vi "Main.vi"(8 "error in (no error)":errorcluster, 11 "ImageStackBase in":refnum<class "ImageStack.lvclass">) -> (0 "error out":errorcluster, 3 "component":refnum<class "ImageStack.lvclass">)   [LabVIEW 2012, in "ImageStack.lvclass"]
doc: "Main VI of the component."
uses:
  ImageStack.lvclass
  <vilib>/Distrio/Murmex/Murmex/command_enum.ctl
  ImageStack.lvclass/ImageStack.ctl
  <vilib>/Distrio/Murmex/InitialiseMessage/InitialiseMessage.lvclass
  <vilib>/Distrio/Murmex/Murmex/data_compression_enum.ctl
  <vilib>/Distrio/Murmex/TerminateMessage/TerminateMessage.lvclass
  <vilib>/Distrio/Murmex/ConfigureMessage/ConfigureMessage.lvclass
  <vilib>/Distrio/Murmex/Murmex/update_cluster.ctl
  <vilib>/Distrio/Murmex/StartMessage/StartMessage.lvclass
  <vilib>/Distrio/Murmex/StopMessage/StopMessage.lvclass
  <vilib>/Distrio/Murmex/Murmex/Set configure at initialise.vi
  <vilib>/Distrio/Murmex/Murmex/Set log reference.vi
  <vilib>/Distrio/Murmex/Murmex/Set VI reference.vi
  <vilib>/Distrio/Murmex/Murmex/Set relay start stop to observers.vi
  <vilib>/Distrio/Murmex/Murmex/Set data compression.vi
  <vilib>/Distrio/Murmex/Murmex/Set write log to disk.vi
  <vilib>/Distrio/Murmex/Murmex/Murmex.lvclass
  <vilib>/Distrio/Murmex/Message/Message.lvclass
panel:
  in  "button:config":bool
  in  "Tab Control":enum32{"User", "Debug", "About"}(tab)
  in  "button::direction":bool
  in  "File name":string
  out "Translation speed":dbl[unit]
  in  "button:start":bool
  in  "No. of frames":u16=100
  out "Frame rate":dbl[unit]
  in  "Subfolder levels":string[](array[string])
  in  "Step size":dbl[unit]
  out "log":string
  in  "ID":string="stack"
  in  "wait b4 acquisition":dbl[unit]=1.0
  in  "button:send command":bool
  in  "Generic command":string
  in  "command":T1
  in  "button:quit":bool
  in  "terminate?":bool=TRUE
  # "ImageStack\n\nImplemented by:\nLudovico Silvestri\nUniversity of Florence, Italy"
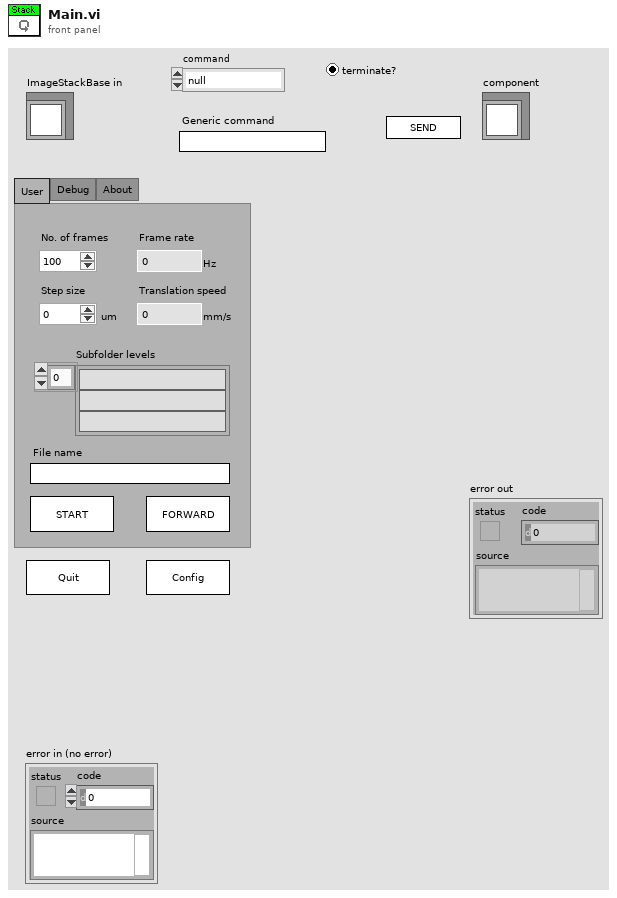
[diagram p1: front panel]
types:
  T1 = typedef "Murmex.lvlib/Murmex.lvclass/command_enum.ctl" = enum16{"null", "initialise", "reset", "terminate", "acknowledge", "update", "inspect", "inform", "proceed", "start", "stop", "fetch", "configure", "generic"}
  T2 = typedef "Murmex.lvlib/Murmex.lvclass/data_compression_enum.ctl" = enum16{"base64", "zip+base64", "byte to string"}
  T3 = typedef "Murmex.lvlib/Murmex.lvclass/update_cluster.ctl" = cluster{"target ID":string, "key chains":string[], "values":variant[]}
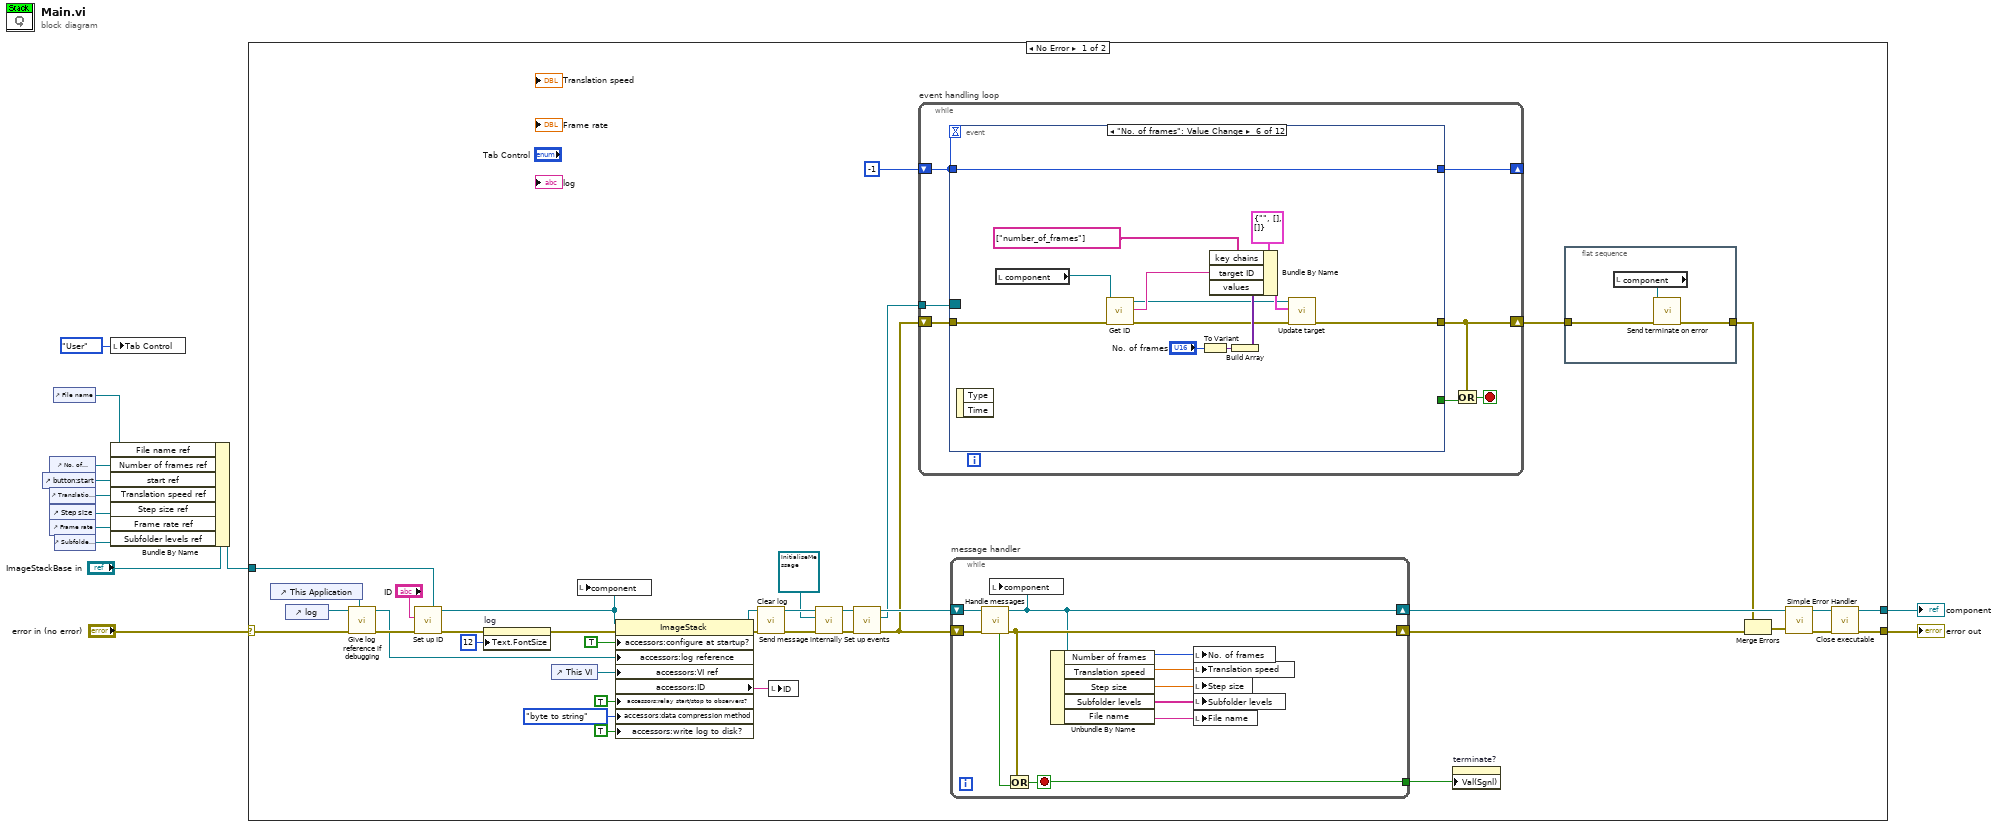
[diagram p0: block diagram]
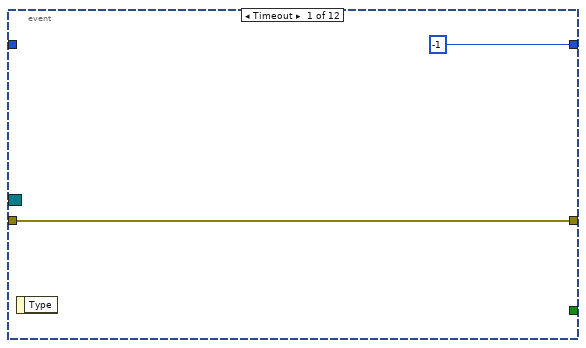
[diagram p2: hidden frame]
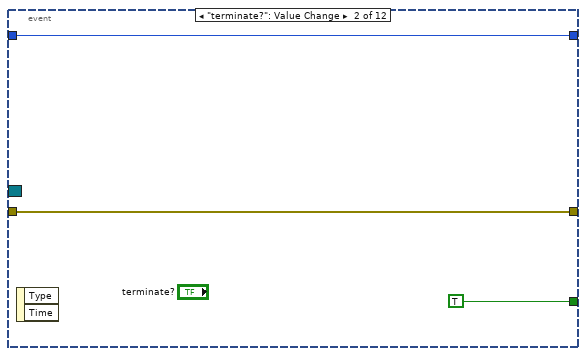
[diagram p3: hidden frame]
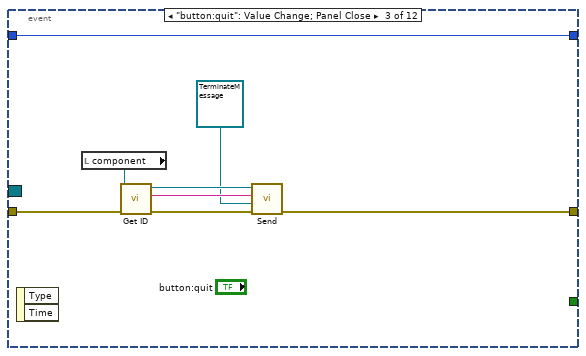
[diagram p4: hidden frame]
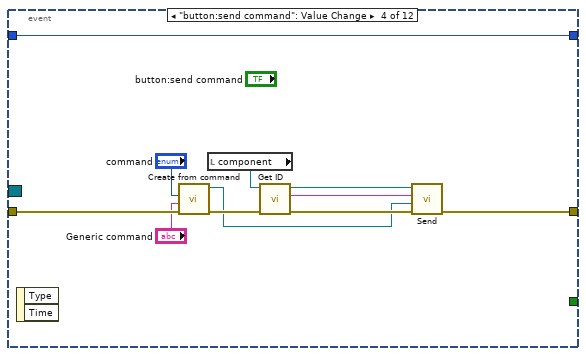
[diagram p5: hidden frame]
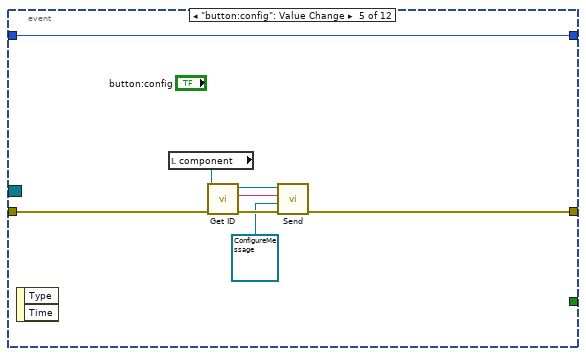
[diagram p6: hidden frame]
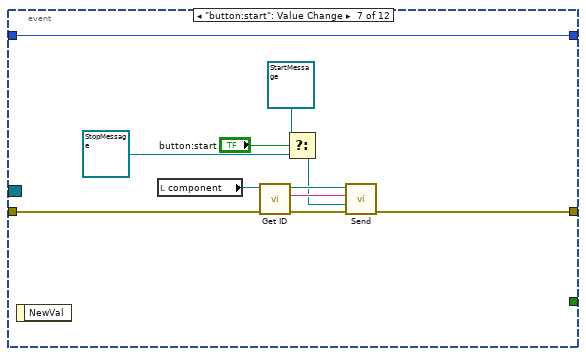
[diagram p7: hidden frame]
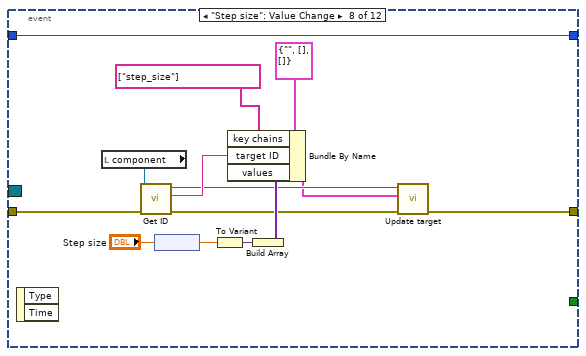
[diagram p8: hidden frame]
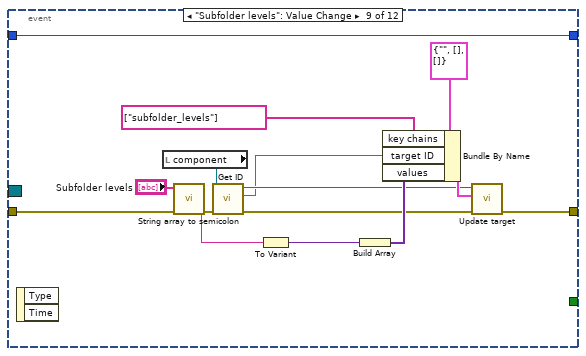
[diagram p9: hidden frame]
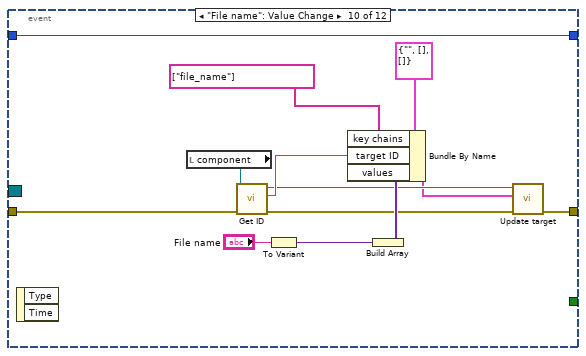
[diagram p10: hidden frame]
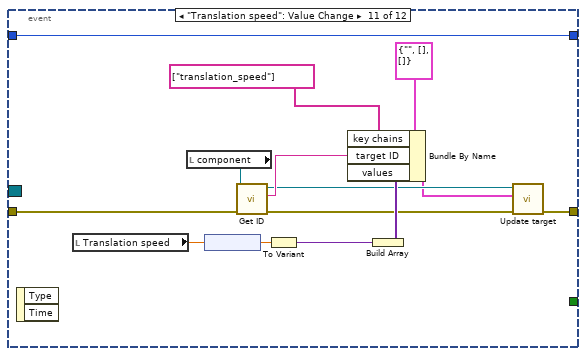
[diagram p11: hidden frame]
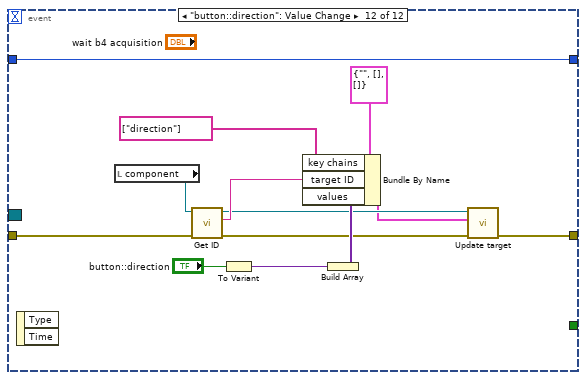
[diagram p12: hidden frame]
diagram:
  n1 = control-ref of="button:start"() -> (w4:refnum<vi>)
  n2 = control-ref of="No. of frames"() -> (w3:refnum<vi>)
  n3 = control-ref of="Translation speed"() -> (w5:refnum<vi>)
  n4 = control-ref of="Step size"() -> (w6:refnum<vi>)
  n5 = control-ref of="Frame rate"() -> (w7:refnum<vi>)
  n6 = control-ref of="File name"() -> (w1:refnum<vi>)
  n7 = control-ref of="Subfolder levels"() -> (w8:refnum<vi>)
  n8 = local write "Tab Control"(enum32{"User", "Debug", "About"}."User" ("Tab Control")) -> ()
  n9 = Bundle By Name(cluster="ImageStackBase in", "File name ref"=w1, "Number of frames ref"=w3, "start ref"=w4, "Translation speed ref"=w5, "Step size ref"=w6, "Frame rate ref"=w7, "Subfolder levels ref"=w8) -> (w9:refnum<class "ImageStack.lvclass">)
  n10 = case shown="No Error" "error in (no error)" {
    selector: "error in (no error)" -> [w19 w197]
    tunnel: w9 -> [w43 w198]
    tunnel: [w22 w198] -> w11
    tunnel: [w23 w197] -> w10
    frame No Error {
      n11 = control-ref of="This Application"() -> (w16:refnum<vi>)
      n12 = control-ref of="log"() -> (w15:refnum<vi>)
      n13 = call "Give log reference if debugging.vi"("application ref"=w16, "error in (no error)"=w19, "log reference in"=w15) -> ("error out"=w18:errorcluster, "log reference out"=w14:refnum<vi>)  [unwired: 6 in, 1 out]
      n14 = call <vilib>:"Set up ID.vi"("error in (no error)"=w18, "component ID"="ID", "MurmexBase in"=w43) -> ("error out"=w32:errorcluster, "MurmexBase out"=w40:refnum<class "ImageStack.lvclass">)  [unwired: 6 in, 1 out]
      n15 = property on="log" class="Str"(error in=w32, "Text.FontSize"=u32 12 ("Text.Font:Size")) -> (error out=w31:errorcluster)  [unwired: 1 in, 1 out]
      n16 = control-ref of="This VI"() -> (w49:refnum<vi>)
      n17 = local write "component"(w40) -> ()
      n18 = property class="ImageStack"(reference=w40, error in=w31, "accessors:configure at startup?"=TRUE ("configure at startup?"), "accessors:log reference"=w14, "accessors:VI ref"=w49, "accessors:relay start/stop to observers?"=TRUE ("relay start/stop to observers?"), "accessors:data compression method"=data_compression_enum."byte to string" ("data compression method"), "accessors:write log to disk?"=TRUE ("write log to disk?")) -> (reference out=w48:refnum<class "ImageStack.lvclass">, error out=w47:errorcluster, "accessors:ID"=w41:string)
      n19 = call <vilib>:"Clear log.vi"("error in (no error)"=w47, "MurmexBase in"=w48) -> ("error out"=w46:errorcluster, "MurmexBase out"=w45:refnum<class "ImageStack.lvclass">)  [unwired: 8 in]
      n20 = local write "ID"(w41) -> ()
      n21 = call <vilib>:"Send message internally.vi"("error in (no error)"=w46, "Message"=refnum<class "InitialiseMessage.lvclass"> refnum ("Murmex.lvlib:InitialiseMessage"), "Murmex in"=w45) -> ("error out"=w39:errorcluster, "Murmex out"=w38:refnum<class "ImageStack.lvclass">)  [unwired: 7 in]
      n22 = call <vilib>:"Set up events.vi"("error in (no error)"=w39, "MurmexBase in"=w38) -> ("error out"=w35:errorcluster, "Event Registration Refnum"=w34:refnum<event-registration>, "MurmexBase out"=w37:refnum<class "ImageStack.lvclass">)  [unwired: 7 in]
      n23 = while "event handling loop" {
        shift-right: [w59] -> _
        shift-left: -1 -> [w60]
        shift-right: [w55] -> w25
        shift-left: w35 -> [w58]
        tunnel: w34 -> [w57]
        stop <- w56 stop-if-true
        n24 = event shown="[5] \"No. of frames\": Value Change" {
          selector: w57 -> [_ _ _ _ _ _ _ _ _ _ _ _]
          dyn-events: _ -> [_ _ _ _ _ _ _ _ _ _ _ _]
          timeout: w60 -> [_ _ _ _ _ _ _ _ _ _ _ _]
          tunnel: w60 -> [_ w63 w66 w74 w85 w101 w106 w118 w140 w148 w162 w173]
          tunnel: [-1 w63 w66 w74 w85 w101 w106 w118 w140 w148 w162 w173] -> w59
          tunnel: [w61 w65 w69 w79 w90 w102 w111 w122 w141 w151 w165 w175] -> w55
          tunnel: w58 -> [w61 w65 w73 w84 w92 w104 w112 w128 w139 w147 w161 w177]
          tunnel: [_ TRUE _ _ _ _ _ _ _ _ _ _] -> w54
          event Timeout {
            n25 = event-data() -> ()  [unwired: 1 in, 1 out]
          }
          event "terminate?": Value Change {
            n26 = event-data() -> ()  [unwired: 1 in, 2 out]
          }
          event "button:quit": Value Change; Panel Close {
            n27 = event-data() -> ()  [unwired: 1 in, 2 out]
            n28 = local read "component"() -> (w72:refnum<class "ImageStack.lvclass">)
            n29 = call <vilib>:"Get ID.vi"("error in (no error)"=w73, "Murmex in"=w72) -> ("error out"=w70:errorcluster, "component id"=w68:string, "Murmex out"=w71:refnum<class "ImageStack.lvclass">)  [unwired: 7 in]
            n30 = call <vilib>:"Send.vi"("error in (no error)"=w70, "Message"=refnum<class "TerminateMessage.lvclass"> refnum ("Murmex.lvlib:TerminateMessage"), "recipient"=w68, "Murmex in"=w71) -> ("error out"=w69:errorcluster)  [unwired: 6 in, 1 out]
          }
          event "button:send command": Value Change {
            n31 = event-data() -> ()  [unwired: 1 in, 2 out]
            n32 = call <vilib>:"Create from command.vi"("error in (no error)"=w84, "generic command"="Generic command", "command"="command") -> ("error out"=w81:errorcluster, "Message out"=w78:refnum<class "Message.lvclass">)  [unwired: 7 in]
            n33 = local read "component"() -> (w77:refnum<class "ImageStack.lvclass">)
            n34 = call <vilib>:"Get ID.vi"("error in (no error)"=w81, "Murmex in"=w77) -> ("error out"=w80:errorcluster, "component id"=w75:string, "Murmex out"=w76:refnum<class "ImageStack.lvclass">)  [unwired: 7 in]
            n35 = call <vilib>:"Send.vi"("error in (no error)"=w80, "Message"=w78, "recipient"=w75, "Murmex in"=w76) -> ("error out"=w79:errorcluster)  [unwired: 6 in, 1 out]
          }
          event "button:config": Value Change {
            n36 = event-data() -> ()  [unwired: 1 in, 2 out]
            n37 = local read "component"() -> (w86:refnum<class "ImageStack.lvclass">)
            n38 = call <vilib>:"Get ID.vi"("error in (no error)"=w92, "Murmex in"=w86) -> ("error out"=w91:errorcluster, "component id"=w88:string, "Murmex out"=w89:refnum<class "ImageStack.lvclass">)  [unwired: 7 in]
            n39 = call <vilib>:"Send.vi"("error in (no error)"=w91, "Message"=refnum<class "ConfigureMessage.lvclass"> refnum ("Murmex.lvlib:ConfigureMessage"), "recipient"=w88, "Murmex in"=w89) -> ("error out"=w90:errorcluster)  [unwired: 6 in, 1 out]
          }
          event "No. of frames": Value Change {
            n40 = event-data() -> ()  [unwired: 1 in, 2 out]
            n41 = local read "component"() -> (w103:refnum<class "ImageStack.lvclass">)
            n42 = call <vilib>:"Get ID.vi"("error in (no error)"=w104, "Murmex in"=w103) -> ("error out"=w93:errorcluster, "component id"=w95:string, "Murmex out"=w94:refnum<class "ImageStack.lvclass">)  [unwired: 7 in]
            n43 = To Variant(anything="No. of frames") -> (Variant=w98:variant)
            n44 = Build Array(w98) -> (w97:variant[])
            n45 = Bundle By Name(cluster=T3 {"target ID"="", "key chains"=[], "values"=[]} ("update cluster"), "key chains"=string[] ["number_of_frames"], "target ID"=w95, "values"=w97) -> (w96:T3)
            n46 = call <vilib>:"Update target.vi"("error in (no error)"=w93, "update cluster"=w96, "MurmexBase in"=w94) -> ("error out"=w102:errorcluster)  [unwired: 7 in, 1 out]
          }
          event "button:start": Value Change {
            n47 = event-data() -> ()  [unwired: 1 in, 1 out]
            n48 = local read "component"() -> (w113:refnum<class "ImageStack.lvclass">)
            n49 = call <vilib>:"Get ID.vi"("error in (no error)"=w112, "Murmex in"=w113) -> ("error out"=w116:errorcluster, "component id"=w114:string, "Murmex out"=w115:refnum<class "ImageStack.lvclass">)  [unwired: 7 in]
            n50 = Select(t=refnum<class "StartMessage.lvclass"> refnum ("Message in"), s="button:start", f=refnum<class "StopMessage.lvclass"> refnum ("Distrio Murmex 1.0:StopMessage")) -> (s? t:f=w108:refnum<class "Message.lvclass">)
            n51 = call <vilib>:"Send.vi"("error in (no error)"=w116, "Message"=w108, "recipient"=w114, "Murmex in"=w115) -> ("error out"=w111:errorcluster)  [unwired: 6 in, 1 out]
          }
          event "Step size": Value Change {
            n52 = event-data() -> ()  [unwired: 1 in, 2 out]
            n53 = local read "component"() -> (w124:refnum<class "ImageStack.lvclass">)
            n54 = call <vilib>:"Get ID.vi"("error in (no error)"=w128, "Murmex in"=w124) -> ("error out"=w123:errorcluster, "component id"=w127:string, "Murmex out"=w121:refnum<class "ImageStack.lvclass">)  [unwired: 7 in]
            n55 = node("Step size") -> (w117:dbl)
            n56 = To Variant(anything=w117) -> (Variant=w126:variant)
            n57 = Build Array(w126) -> (w125:variant[])
            n58 = Bundle By Name(cluster=T3 {"target ID"="", "key chains"=[], "values"=[]} ("update cluster"), "key chains"=string[] ["step_size"], "target ID"=w127, "values"=w125) -> (w120:T3)
            n59 = call <vilib>:"Update target.vi"("error in (no error)"=w123, "update cluster"=w120, "MurmexBase in"=w121) -> ("error out"=w122:errorcluster)  [unwired: 7 in, 1 out]
          }
          event "Subfolder levels": Value Change {
            n60 = event-data() -> ()  [unwired: 1 in, 2 out]
            n61 = local read "component"() -> (w142:refnum<class "ImageStack.lvclass">)
            n62 = call "String array to semicolon.vi"("error in"=w139, "String array"="Subfolder levels") -> ("error out"=w138:errorcluster, "Semicolon string"=w136:string)  [unwired: 8 in]
            n63 = call <vilib>:"Get ID.vi"("error in (no error)"=w138, "Murmex in"=w142) -> ("error out"=w132:errorcluster, "component id"=w131:string, "Murmex out"=w133:refnum<class "ImageStack.lvclass">)  [unwired: 7 in]
            n64 = To Variant(anything=w136) -> (Variant=w143:variant)
            n65 = Build Array(w143) -> (w135:variant[])
            n66 = Bundle By Name(cluster=T3 {"target ID"="", "key chains"=[], "values"=[]} ("update cluster"), "key chains"=string[] ["subfolder_levels"], "target ID"=w131, "values"=w135) -> (w134:T3)
            n67 = call <vilib>:"Update target.vi"("error in (no error)"=w132, "update cluster"=w134, "MurmexBase in"=w133) -> ("error out"=w141:errorcluster)  [unwired: 7 in, 1 out]
          }
          event "File name": Value Change {
            n68 = event-data() -> ()  [unwired: 1 in, 2 out]
            n69 = local read "component"() -> (w153:refnum<class "ImageStack.lvclass">)
            n70 = call <vilib>:"Get ID.vi"("error in (no error)"=w147, "Murmex in"=w153) -> ("error out"=w152:errorcluster, "component id"=w156:string, "Murmex out"=w150:refnum<class "ImageStack.lvclass">)  [unwired: 7 in]
            n71 = To Variant(anything="File name") -> (Variant=w155:variant)
            n72 = Build Array(w155) -> (w154:variant[])
            n73 = Bundle By Name(cluster=T3 {"target ID"="", "key chains"=[], "values"=[]} ("update cluster"), "key chains"=string[] ["file_name"], "target ID"=w156, "values"=w154) -> (w149:T3)
            n74 = call <vilib>:"Update target.vi"("error in (no error)"=w152, "update cluster"=w149, "MurmexBase in"=w150) -> ("error out"=w151:errorcluster)  [unwired: 7 in, 1 out]
          }
          event "Translation speed": Value Change {
            n75 = event-data() -> ()  [unwired: 1 in, 2 out]
            n76 = local read "Translation speed"() -> (w160:dbl[unit])
            n77 = local read "component"() -> (w167:refnum<class "ImageStack.lvclass">)
            n78 = node(w160) -> (w159:dbl)
            n79 = call <vilib>:"Get ID.vi"("error in (no error)"=w161, "Murmex in"=w167) -> ("error out"=w166:errorcluster, "component id"=w170:string, "Murmex out"=w164:refnum<class "ImageStack.lvclass">)  [unwired: 7 in]
            n80 = To Variant(anything=w159) -> (Variant=w169:variant)
            n81 = Build Array(w169) -> (w168:variant[])
            n82 = Bundle By Name(cluster=T3 {"target ID"="", "key chains"=[], "values"=[]} ("update cluster"), "key chains"=string[] ["translation_speed"], "target ID"=w170, "values"=w168) -> (w163:T3)
            n83 = call <vilib>:"Update target.vi"("error in (no error)"=w166, "update cluster"=w163, "MurmexBase in"=w164) -> ("error out"=w165:errorcluster)  [unwired: 7 in, 1 out]
          }
          event "button::direction": Value Change {
            n84 = event-data() -> ()  [unwired: 1 in, 2 out]
            n85 = local read "component"() -> (w176:refnum<class "ImageStack.lvclass">)
            n86 = call <vilib>:"Get ID.vi"("error in (no error)"=w177, "Murmex in"=w176) -> ("error out"=w181:errorcluster, "component id"=w184:string, "Murmex out"=w180:refnum<class "ImageStack.lvclass">)  [unwired: 7 in]
            n87 = To Variant(anything="button::direction") -> (Variant=w183:variant)
            n88 = Build Array(w183) -> (w182:variant[])
            n89 = Bundle By Name(cluster=T3 {"target ID"="", "key chains"=[], "values"=[]} ("update cluster"), "key chains"=string[] ["direction"], "target ID"=w184, "values"=w182) -> (w179:T3)
            n90 = call <vilib>:"Update target.vi"("error in (no error)"=w181, "update cluster"=w179, "MurmexBase in"=w180) -> ("error out"=w175:errorcluster)  [unwired: 7 in, 1 out]
          }
        }
        n91 = Or(x=w55, y=w54) -> (x .or. y?=w56:bool)
      }
      n92 = while "message handler" {
        shift-right: [w191] -> w21
        shift-left: w37 -> [w196]
        shift-right: [w194] -> w24
        shift-left: w35 -> [w195]
        tunnel: [w192] -> w33
        stop <- w192 stop-if-true
        n93 = call <vilib>:"Handle messages.vi"("error in (no error)"=w195, "Murmex in"=w196) -> ("error out"=w194:errorcluster, "Murmex out"=w191:refnum<class "ImageStack.lvclass">, "terminated?"=w193:bool)  [unwired: 7 in]
        n94 = local write "component"(w191) -> ()
        n95 = Or(x=w194, y=w193) -> (x .or. y?=w192:bool)
        n96 = Unbundle By Name(w191) -> ("Number of frames"=w189:u16, "Translation speed"=w190:dbl[unit], "Step size"=w188:dbl[unit], "Subfolder levels"=w187:string[], "File name"=w186:string)
        n97 = local write "No. of frames"(w189) -> ()
        n98 = local write "Translation speed"(w190) -> ()
        n99 = local write "Step size"(w188) -> ()
        n100 = local write "Subfolder levels"(w187) -> ()
        n101 = local write "File name"(w186) -> ()
      }
      n102 = property on="terminate?" class="Bool (strict)"("Val(Sgnl)"=w33) -> ()  [unwired: 2 in, 2 out]
      n103 = flat-sequence {
        tunnel: w25 -> [w53]
        tunnel: [w51] -> w20
        frame #0 {
          n104 = local read "component"() -> (w52:refnum<class "ImageStack.lvclass">)
          n105 = call <vilib>:"Send terminate on error.vi"("error in (no error)"=w53, "Murmex in"=w52) -> ("error out"=w51:errorcluster)  [unwired: 8 in, 1 out]
        }
      }
      n106 = Merge Errors(w20, w24) -> (w26:errorcluster)
      n107 = call <vilib>:"Simple Error Handler.vi"("error in (no error)"=w26) -> ("error out"=w27:errorcluster)  [unwired: 4 in, 4 out]
      n108 = call <vilib>:"Close executable.vi"("error in (no error)"=w27, "MurmexBase in"=w21) -> ("error out"=w23:errorcluster, "MurmexBase out"=w22:refnum<class "ImageStack.lvclass">)  [unwired: 8 in]
    }
    frame Error {
    }
  }
  "error out" <- w10
  "component" <- w11
